vi "global for picoscope.vi"() -> ()   [LabVIEW 2024]
panel:
  in  "z cut length bottom":u32
  in  "z cut length top":u32
  in  "x cut length":u32
  in  "x shift":dbl format="%_3g"
  in  "z shift":dbl format="%_3g"
  in  "am2":dbl
  in  "round-trip anal":bool
  in  "round-trip":bool
  in  "fit coeffs":dbl[][](array[numeric])
  in  "am":dbl
  in  "ao1":dbl
  in  "Tpp":dbl
  in  "g":dbl
  in  "b":dbl
  in  "Taod":dbl=10.0
  in  "frames to record":i32=10
  in  "frames for calib":i32=10
  in  "calib/monitor":bool
  in  "z pixel size [um]":dbl=10.0
  in  "g2 period [us]":dbl
  in  "monitor 2D":bool
  in  "Nx":dbl
  in  "AOD scan speed ratio":dbl=10.0
  in  "dead time for burst [us]":dbl=10.0
  in  "ofst for g1":dbl=10.0
  in  "ofst for g2":dbl=10.0
  in  "pixel size [um] P":dbl=10.0
  in  "g2 voltage to disp. at img. [um/V]":dbl
  in  "g1 voltage to disp. at obj. [um/V]":dbl
  in  "phase for g2":dbl
  in  "Vpp2 adj":dbl
  in  "Vpp1 adj":dbl
  in  "Nzf":i32=10
  in  "Nv":i32=3
  in  "samples [us]":u32=2000
  in  "trig delay [us]":u32=200
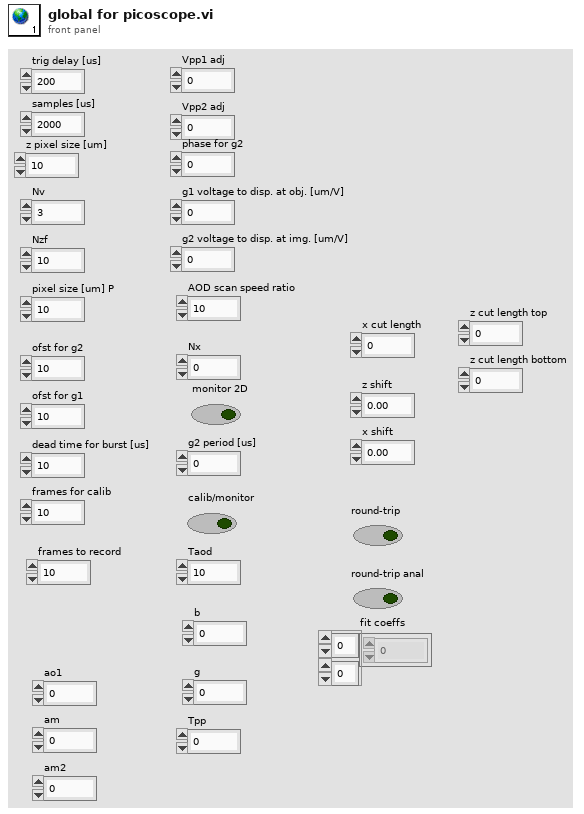
[diagram p1: front panel]
diagram:
